vi "Evaluate Part 1.vi"() -> ()   [LabVIEW 2021]
uses:
  Proto/Proto.lvclass
panel:
  out "Load":u64
  in  "Input":string="O....#....\nO.OO#....#\n.....##...\nOO.#O....O\n.O.....O#.\nO.#..O.#.#\n..O..#O..O\n.......O..\n#....###..\n#OO..#...."
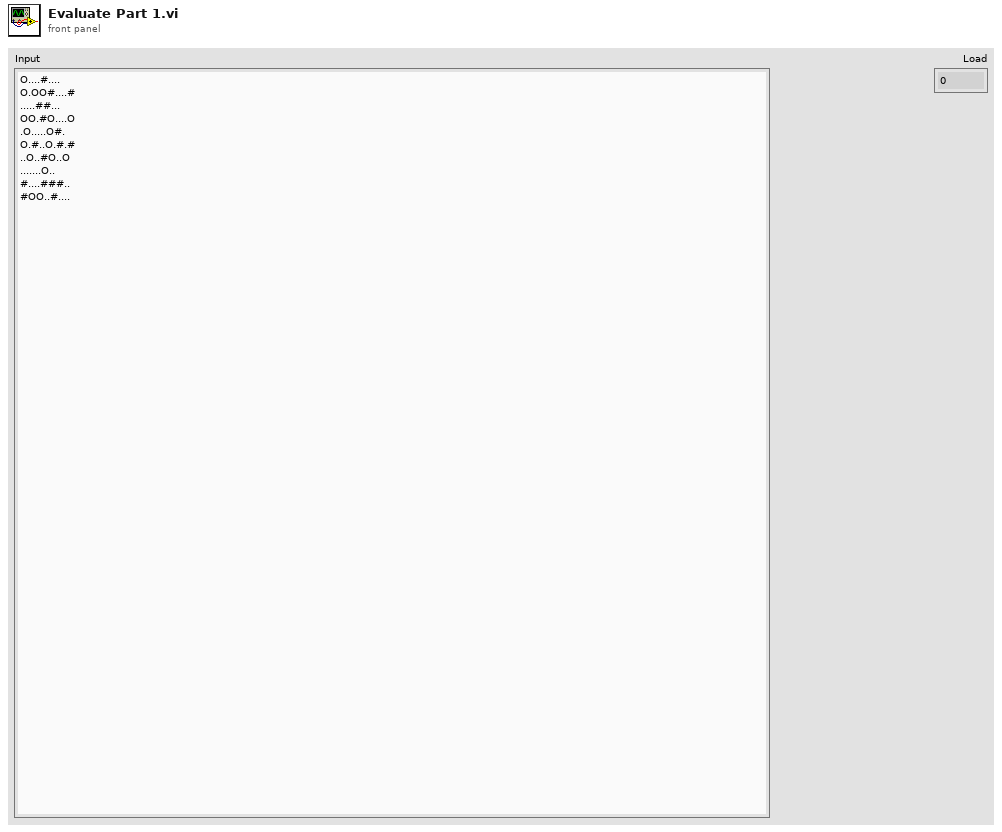
[diagram p1: front panel]
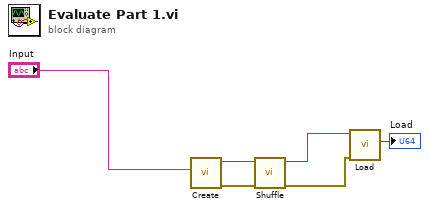
[diagram p0: block diagram]
diagram:
  n1 = call "Create.vi"("Input"="Input") -> ("error out"=w6:errorcluster, "Proto"=w5:refnum<class "Proto.lvclass">)  [unwired: 9 in]
  n2 = call "Shuffle.vi"("error in (no error)"=w6, "Proto in"=w5) -> ("error out"=w3:errorcluster, "Proto out"=w2:refnum<class "Proto.lvclass">)  [unwired: 8 in]
  n3 = call "Load.vi"("error in (no error)"=w3, "Proto in"=w2) -> ("Load"=→"Load":u64)  [unwired: 7 in, 2 out]
